vi "Normal CDF.vi"(9 "std":dbl=1.0, 10 "mean":dbl, 11 "x":dbl) -> (0 "error":i32, 3 "cdf(x)":dbl=0.5 format="%.6g")   [LabVIEW 2017, in "NI_Gmath.lvlib"]
doc: "Computes the continuous cumulative distribution function (CDF), or the probability that the random variate X, where X describes the selected distribution type, has a value less than or equal to <B>x</B>. You must manually select the polymorphic instance to use."
uses:
  NI_Gmath.lvlib
  st_error_code.ctl
panel:
  # "Normal CDF"
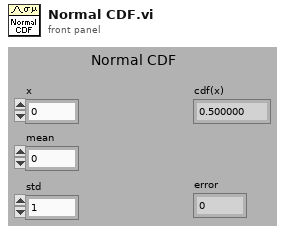
[diagram p1: front panel]
types:
  T1 = typedef "NI_Gmath.lvlib/st_error_code.ctl" = i32
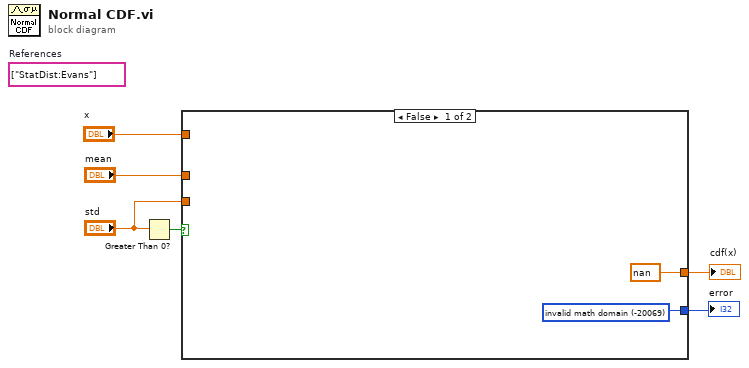
[diagram p0: block diagram]
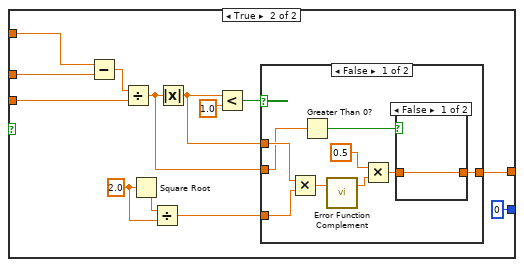
[diagram p2: hidden frame]
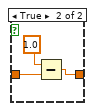
[diagram p3: hidden frame]
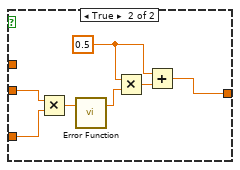
[diagram p4: hidden frame]
diagram:
  (unwired) string[] ["StatDist:Evans"]  # References
  n1 = Greater Than 0?(x="std") -> (x > 0?=w6:bool)
  n2 = case shown="False" w6 {
    tunnel: "std" -> [_ w17]
    tunnel: [w7 0 ("invalid math domain")] -> w4
    tunnel: [nan w10] -> w3
    tunnel: "x" -> [_ w9]
    tunnel: "mean" -> [_ w20]
    frame False {
      w7 = T1 -20069 items=["invalid math domain"=-20069, "Fourier interpolation size m >= n"=-20070, "empty array"=-20003] ("stat interp error code")
    }
    frame True {
      w18 = 2.0
      n3 = Subtract(x=w9, y=w20) -> (x-y=w16:dbl)
      n4 = Divide(x=w16, y=w17) -> (x/y=w13:dbl)
      n5 = Square Root(x=w18) -> (sqrt(x)=w19:dbl)
      n6 = Divide(x=w19, y=w18) -> (x/y=w12:dbl)
      n7 = Absolute Value(x=w13) -> (abs(x)=w11:dbl)
      n8 = Less?(x=w11, y=1.0) -> (x < y?=w14:bool)
      n9 = case shown="False" w14 {
        tunnel: w13 -> [w25 w40]
        tunnel: w12 -> [w26 w41]
        tunnel: [w22 w35] -> w10
        tunnel: w11 -> [w27 _]
        frame False {
          n10 = Multiply(x=w27, y=w26) -> (x*y=w30:dbl)
          n11 = Greater Than 0?(x=w25) -> (x > 0?=w24:bool)
          n12 = call "Error Function Complement.vi"("x"=w30) -> ("1 - erf(x)"=w29:dbl)  [unwired: 2 in]
          n13 = Multiply(x=0.5, y=w29) -> (x*y=w23:dbl)
          n14 = case shown="False" w24 {
            tunnel: w23 -> [w31 w33]
            tunnel: [w31 w32] -> w22
            frame False {
            }
            frame True {
              n15 = Subtract(x=1.0, y=w33) -> (x-y=w32:dbl)
            }
          }
        }
        frame True {
          w36 = 0.5
          n16 = Multiply(x=w40, y=w41) -> (x*y=w39:dbl)
          n17 = call "Error Function.vi"("x"=w39) -> ("erf(x)"=w38:dbl)  [unwired: 2 in]
          n18 = Multiply(x=w36, y=w38) -> (x*y=w37:dbl)
          n19 = Add(x=w36, y=w37) -> (x+y=w35:dbl)
        }
      }
    }
  }
  "cdf(x)" <- w3
  "error" <- w4
